vi "ConfigUtilities - Update Properties.vi"(4 "Channel Data Types":string[](array[string]), 6 "Tx?":bool, 8 "error in (no error)":errorcluster, 9 "Channel Paths":string[](array[string]), 10 "Channel Names":string[](array[string]), 11 "Item Ref in":T1 format="%.0x") -> (0 "error out":errorcluster, 3 "Item Ref out":T1=18446744073709551615 format="%.0x")   [LabVIEW 2016, in "UDP-Custom-Device System Explorer.lvlib"]
uses:
  UDP-Custom-Device System Explorer.lvlib
  <vilib>/NI Veristand/Custom Device API/Custom Device Item Ref.ctl
  Shared/Constants.vi
  <vilib>/NI Veristand/Custom Device API/Set Item Property (String Array).vi
  <vilib>/NI VeriStand/Custom Device API/Custom Device API.lvlib
  <vilib>/NI VeriStand/Custom Device Tools/Custom Device Utility Library/Custom Device Utility Library.lvlib
  Shared/UDP-Custom-Device Shared.lvlib
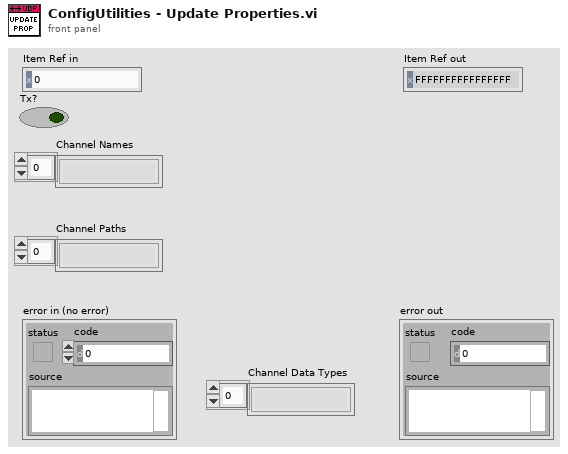
[diagram p1: front panel]
types:
  T1 = typedef "Custom Device API.lvlib/Custom Device Item Ref.ctl" = u64
  T2 = typedef "UDP-Custom-Device Shared.lvlib/Channel Data Type.ctl" = enum16{"Boolean", "Single"}
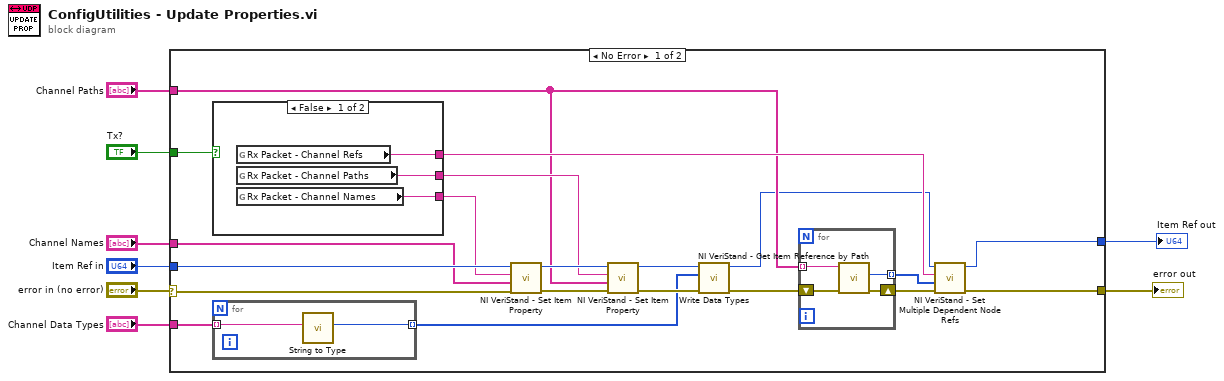
[diagram p0: block diagram]
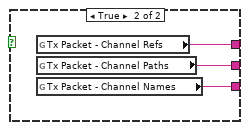
[diagram p2: hidden frame]
diagram:
  n1 = case shown="No Error" "error in (no error)" {
    selector: "error in (no error)" -> [w17 w42]
    tunnel: [w27 w42] -> w8
    tunnel: "Item Ref in" -> [w23 w41]
    tunnel: [w22 w41] -> w6
    tunnel: "Tx?" -> [w18 _]
    tunnel: "Channel Data Types" -> [w10 _]
    tunnel: "Channel Paths" -> [w16 _]
    tunnel: "Channel Names" -> [w15 _]
    frame No Error {
      n2 = case shown="False" w18 {
        tunnel: [w33 w35] -> w21
        tunnel: [w32 w34] -> w20
        tunnel: [w31 w36] -> w19
        frame False {
          n3 = global read "Constants.vi" "Rx Packet - Channel Refs"() -> (w31:string)
          n4 = global read "Constants.vi" "Rx Packet - Channel Paths"() -> (w32:string)
          n5 = global read "Constants.vi" "Rx Packet - Channel Names"() -> (w33:string)
        }
        frame True {
          n6 = global read "Constants.vi" "Tx Packet - Channel Refs"() -> (w36:string)
          n7 = global read "Constants.vi" "Tx Packet - Channel Paths"() -> (w34:string)
          n8 = global read "Constants.vi" "Tx Packet - Channel Names"() -> (w35:string)
        }
      }
      n9 = for {
        tunnel: w10 -> [w30] mode=indexing
        tunnel: [w29] -> w9 mode=indexing
        n10 = call "String to Type.vi"("String Type"=w30) -> ("Data Type"=w29:T2)  [unwired: 10 in]
      }
      n11 = call-poly <vilib>:"NI VeriStand - Set Item Property.vi"("error in (no error)"=w17, "Value"=w15, "Property Name"=w21, "Item Ref in"=w23) -> ("error out"=w24:errorcluster, "Item Ref out"=w25:T1)  [unwired: 5 in, 1 out]
      n12 = call-poly <vilib>:"NI VeriStand - Set Item Property.vi"("error in (no error)"=w24, "Value"=w16, "Property Name"=w20, "Item Ref in"=w25) -> ("error out"=w12:errorcluster, "Item Ref out"=w14:T1)  [unwired: 5 in, 1 out]
      n13 = call "Write Data Types.vi"("error in (no error)"=w12, "Data Types"=w9, "Node Ptr"=w14) -> ("error out"=w11:errorcluster, "Node Ptr out"=w13:T1)  [unwired: 7 in]
      n14 = for {
        shift-right: [w39] -> w28
        shift-left: w11 -> [w40]
        tunnel: w16 -> [w38] mode=indexing
        tunnel: [w37] -> w26 mode=indexing
        n15 = call <vilib>:"NI VeriStand - Get Item Reference by Path.vi"("error in (no error)"=w40, "Item Path in"=w38) -> ("error out"=w39:errorcluster, "Item Ref"=w37:T1)  [unwired: 6 in, 2 out]
      }
      n16 = call <vilib>:"NI VeriStand - Set Multiple Dependent Node Refs.vi"("error in (no error)"=w28, "Dependent Node Refs"=w26, "Base Property Name"=w19, "Item Ref in"=w13) -> ("error out"=w27:errorcluster, "Item Ref out"=w22:T1)  [unwired: 6 in]
    }
    frame Error {
    }
  }
  "error out" <- w8
  "Item Ref out" <- w6
